vi "Page_Windows_Security_Read.vi"(6 "ctlReferences":T1, 8 "error in (no error)":errorcluster, 11 "AB_Application in":refnum<class "AB_Application.lvclass">) -> (0 "error out":errorcluster, 3 "AB_Application out":refnum<class "AB_Application.lvclass">)   [LabVIEW 2020, in "AB_Application.lvclass"]
uses:
  <vilib>/AppBuilder/AB_Classes/Application/AB_Application.lvclass
  <resource>/Framework/Providers/Builds/AppBuilder/AB_UI_Page_Windows_Security_References.ctl
  <resource>/Framework/Providers/Common/provcom_BrowseProjectFile.ctl
  <vilib>/AppBuilder/AB_Classes/Application/AB_Application.lvclass/AB_Application.ctl
  <resource>/Framework/Providers/Common/provcom_StringGlobals.vi
  <vilib>/AppBuilder/CodeSignAPI/CodeSignAPI.lvlib
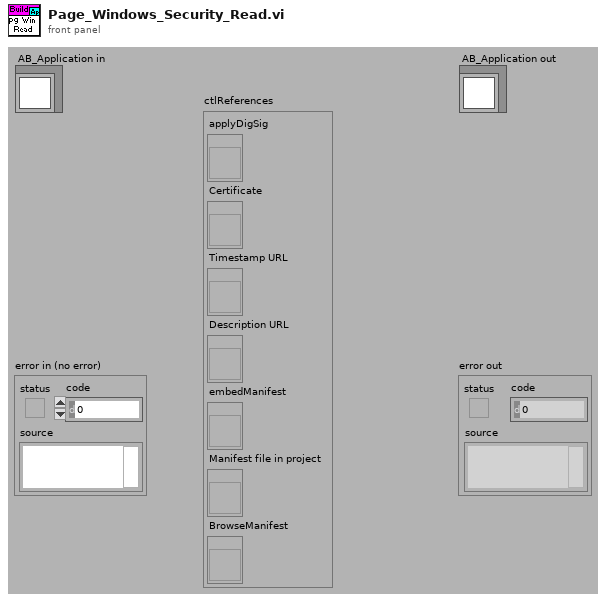
[diagram p1: front panel]
types:
  T1 = typedef "AB_UI_Page_Windows_Security_References.ctl" = cluster{"applyDigSig":refnum<vi>, "Certificate":refnum<vi>, "Timestamp URL":refnum<vi>, "Description URL":refnum<vi>, "embedManifest":refnum<vi>, "Manifest file in project":refnum<vi>, "BrowseManifest":refnum<vi>}
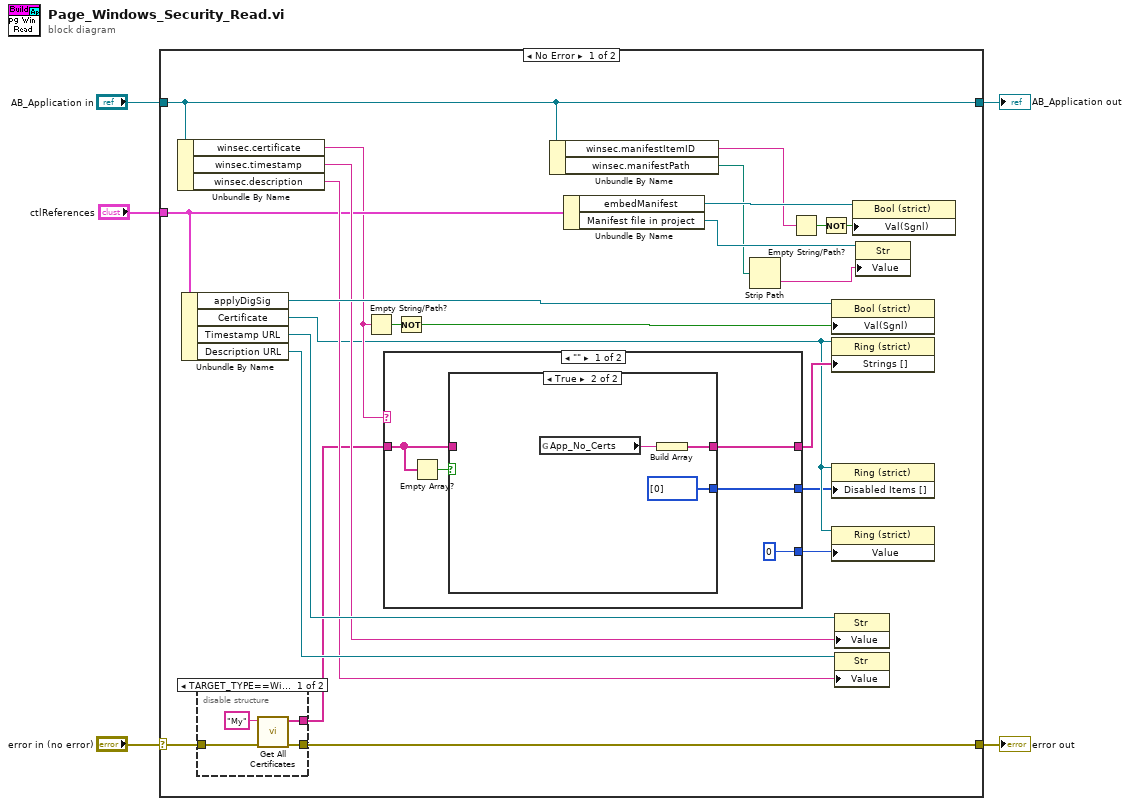
[diagram p0: block diagram]
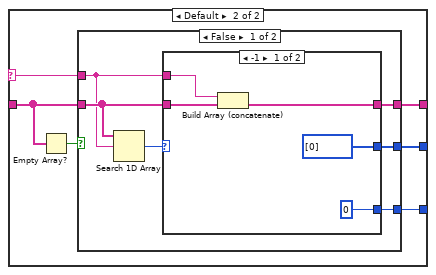
[diagram p4: hidden frame]
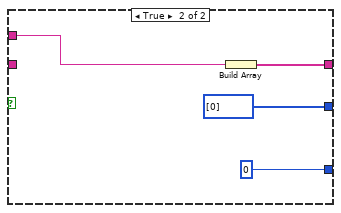
[diagram p6: hidden frame]
diagram:
  n1 = case shown="No Error" "error in (no error)" {
    selector: "error in (no error)" -> [w29 w67]
    tunnel: "AB_Application in" -> [w22 w68]
    tunnel: [w22 w68] -> w3
    tunnel: [w28 w67] -> w2
    tunnel: "ctlReferences" -> [w21 _]
    frame No Error {
      n2 = Unbundle By Name(w22) -> ("winsec.certificate"=w16:string, "winsec.timestamp"=w25:string, "winsec.description"=w23:string)
      n3 = Unbundle By Name(w21) -> ("applyDigSig"=w27:refnum<vi>, "Certificate"=w12:refnum<vi>, "Timestamp URL"=w26:refnum<vi>, "Description URL"=w24:refnum<vi>)
      n4 = disable-structure shown="TARGET_TYPE==Windows" {
        disable-tunnel: w29 -> [w32 w34]
        disable-tunnel: [w31 w34] -> w28
        disable-tunnel: [w30 _] -> w15
        frame condition #0 (active) {
          n5 = call <vilib>:"Get All Certificates.vi"("error in (no error)"=w32, "store"="My") -> ("error out"=w31:errorcluster, "Certificates"=w30:string[])  [unwired: 8 out]
        }
        frame condition #1 {
        }
      }
      n6 = Empty String/Path?(string/path=w16) -> (empty?=w18:bool)
      n7 = case shown="\"\"" w16 {
        selector: w16 -> [_ w46]
        tunnel: w15 -> [w38 w48]
        tunnel: [w37 w45] -> w14
        tunnel: [u16 0 ("Value") w47] -> w13
        tunnel: [w35 w44] -> w11
        frame "" {
          n8 = Empty Array?(array=w38) -> (empty?=w39:bool)
          n9 = case shown="True" w39 {
            tunnel: [w40 w42] -> w37
            tunnel: w38 -> [w40 _]
            tunnel: [_ i32[] [0]] -> w35
            frame False {
            }
            frame True {
              n10 = global read "provcom_StringGlobals.vi" "App_No_Certs"() -> (w43:string)
              n11 = Build Array(w43) -> (w42:string[])
            }
          }
        }
        frame Default {
          n12 = Empty Array?(array=w48) -> (empty?=w49:bool)
          n13 = case shown="False" w49 {
            tunnel: [w53 w66] -> w45
            tunnel: w48 -> [w54 _]
            tunnel: [w50 0] -> w47
            tunnel: w46 -> [w52 w64]
            tunnel: [w51 i32[] [0]] -> w44
            frame False {
              n14 = Search 1D Array(1D array=w54, element=w52) -> (index of element=w55:i32)  [unwired: 1 out]
              n15 = case shown="-1" w55 {
                selector: w55 -> [_ w61]
                tunnel: [w56 w62] -> w53
                tunnel: w54 -> [w60 w62]
                tunnel: w52 -> [w59 _]
                tunnel: [i32[] [0] _] -> w51
                tunnel: [0 w61] -> w50
                frame -1 {
                  n16 = Build Array (concatenate)(w59, w60) -> (w56:string[])
                }
                frame Default {
                }
              }
            }
            frame True {
              n17 = Build Array(w64) -> (w66:string[])
            }
          }
        }
      }
      n18 = Not(x=w18) -> (.not. x?=w17:bool)
      n19 = Unbundle By Name(w22) -> ("winsec.manifestItemID"=w8:string, "winsec.manifestPath"=w7:path)
      n20 = Unbundle By Name(w21) -> ("embedManifest"=w20:refnum<vi>, "Manifest file in project"=w19:refnum<vi>)
      n21 = Strip Path(path=w7) -> (name=w6:string)  [unwired: 1 out]
      n22 = Empty String/Path?(string/path=w8) -> (empty?=w10:bool)
      n23 = Not(x=w10) -> (.not. x?=w9:bool)
      n24 = property class="Bool (strict)"(reference=w27, "Val(Sgnl)"=w17) -> ()  [unwired: 1 in, 2 out]
      n25 = property class="Ring (strict)"(reference=w12, "Strings []"=w14) -> ()  [unwired: 1 in, 2 out]
      n26 = property class="Ring (strict)"(reference=w12, "Disabled Items []"=w11) -> ()  [unwired: 1 in, 2 out]
      n27 = property class="Ring (strict)"(reference=w12, "Value"=w13) -> ()  [unwired: 1 in, 2 out]
      n28 = property class="Str"(reference=w26, "Value"=w25) -> ()  [unwired: 1 in, 2 out]
      n29 = property class="Str"(reference=w24, "Value"=w23) -> ()  [unwired: 1 in, 2 out]
      n30 = property class="Bool (strict)"(reference=w20, "Val(Sgnl)"=w9) -> ()  [unwired: 1 in, 2 out]
      n31 = property class="Str"(reference=w19, "Value"=w6) -> ()  [unwired: 1 in, 2 out]
    }
    frame Error {
    }
  }
  "error out" <- w2
  "AB_Application out" <- w3
